vi "Set TargetTorque.vi"(8 "error in (no error)":errorcluster, 11 "Value":sgl=9.0) -> (0 "error out":errorcluster)   [LabVIEW 2020, in "输出轴伺服.lvlib"]
uses:
  Servo_global.vi
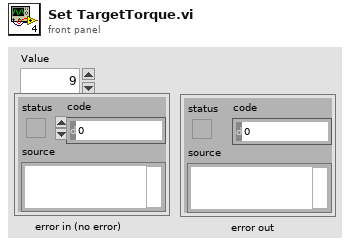
[diagram p1: front panel]
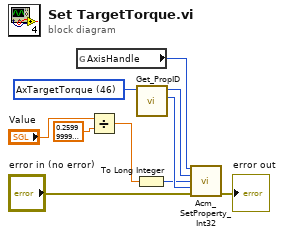
[diagram p0: block diagram]
diagram:
  w10 = u16 46 items=["AxTargetPosition"=44, "AxTargetVelocity"=45, "AxTargetTorque"=46, "AxControlWord"=47, "AxStatusWord"=48, "AxOperationMode"=49, "AxMaxTorque"=333] ("Prop")
  n1 = global read "Servo_global.vi" "AxisHandle"() -> (w1:u32)
  n2 = Divide(x="Value", y=sgl 0.26) -> (x/y=w7:sgl)
  n3 = To Long Integer(number=w7) -> (32bit integer=w3:i32)
  n4 = call "Get_PropID.vi"("Prop"=w10) -> ("BufferLength"=w4:u32, "PropID"=w2:u32)  [unwired: 9 in]
  n5 = call <userlib>:"Acm_SetProperty_Int32.vi"("Handle"=w1, "ProperyID"=w2, "Buffer"=w3, "BufferLength"=w4, "error in (no error)"="error in (no error)") -> ("error out"=→"error out":errorcluster)  [unwired: 8 in, 2 out]
